vi "Set Analog Read Period.vi"(8 "error in (no error)":errorcluster, 10 "Loop Period in ms (10)":u32, 11 "Analog Reader in":refnum<class "Analog Reader.lvclass">) -> (0 "error out":errorcluster, 3 "Analog Reader out":refnum<class "Analog Reader.lvclass">)   [LabVIEW 2024, in "DAQmx Actor.lvlib" / "Analog Reader.lvclass"]
uses:
  Analog Reader.lvclass
  Analog Reader.lvclass/Analog Reader.ctl
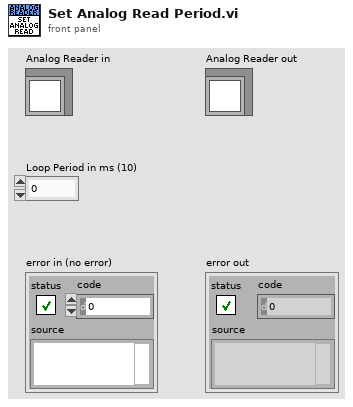
[diagram p1: front panel]
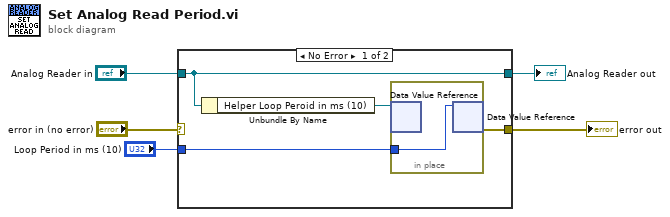
[diagram p0: block diagram]
diagram:
  n1 = case shown="No Error" "error in (no error)" {
    selector: "error in (no error)" -> [_ w12]
    tunnel: [w6 w12] -> w4
    tunnel: [w9 w11] -> w2
    tunnel: "Analog Reader in" -> [w9 w11]
    tunnel: "Loop Period in ms (10)" -> [w7 _]
    frame No Error {
      n2 = Unbundle By Name(w9) -> ("Helper Loop Peroid in ms (10)"=w8:refnum<data-value>)
      n3 = in-place {
        in-place-border: w7 -> [w10]
        n4 = in-place-dvr #1(w8) -> ()  [unwired: 2 out]
        n5 = in-place-dvr #1(w10) -> (w6:errorcluster)  [unwired: 1 out]
      }
    }
    frame Error {
    }
  }
  "error out" <- w4
  "Analog Reader out" <- w2
